vi "Test Filters.vi"() -> ()   [LabVIEW 2019]
uses:
  src/xy_utilities.lvlib
  src/subVIs/Zero Phase Lowpass Filter (multiple).vi
  src/subVIs/Savitsky Golay Weighted Filter (multiple).vi
  src/subVIs/Savitsky Golay Filter (multiple).vi
  src/subVIs/Moving Average (multiple).vi
panel:
  in  "cutoff period (data)":dbl
  in  "Window":dbl
  in  "Window Order":i32
  in  "polynomial order (3)":i32=3
  out "Intensity Graph 2":dbl[][](graph)
  out "Intensity Graph":dbl[][](graph)
  in  "side points":dbl
  in  "Dataset":T1(ring)=enum."superlattice waveguide"
  in  "index":i32
  out "XY Data Filtered 2":cluster{"X-array":dbl[], "Y-array":dbl[]}[](graph)
  in  "Filter":enum16{"Lowpass", "SG", "SGW", "Moving"}(ring)
  out "execution time (s)":dbl
  out "XY Data Filtered":cluster{"X-array":dbl[], "Y-array":dbl[]}[](graph)
  out "XY Data":cluster{"X-array":dbl[], "Y-array":dbl[]}[](graph)
  # "0: 21\"\n5: 0.09\""
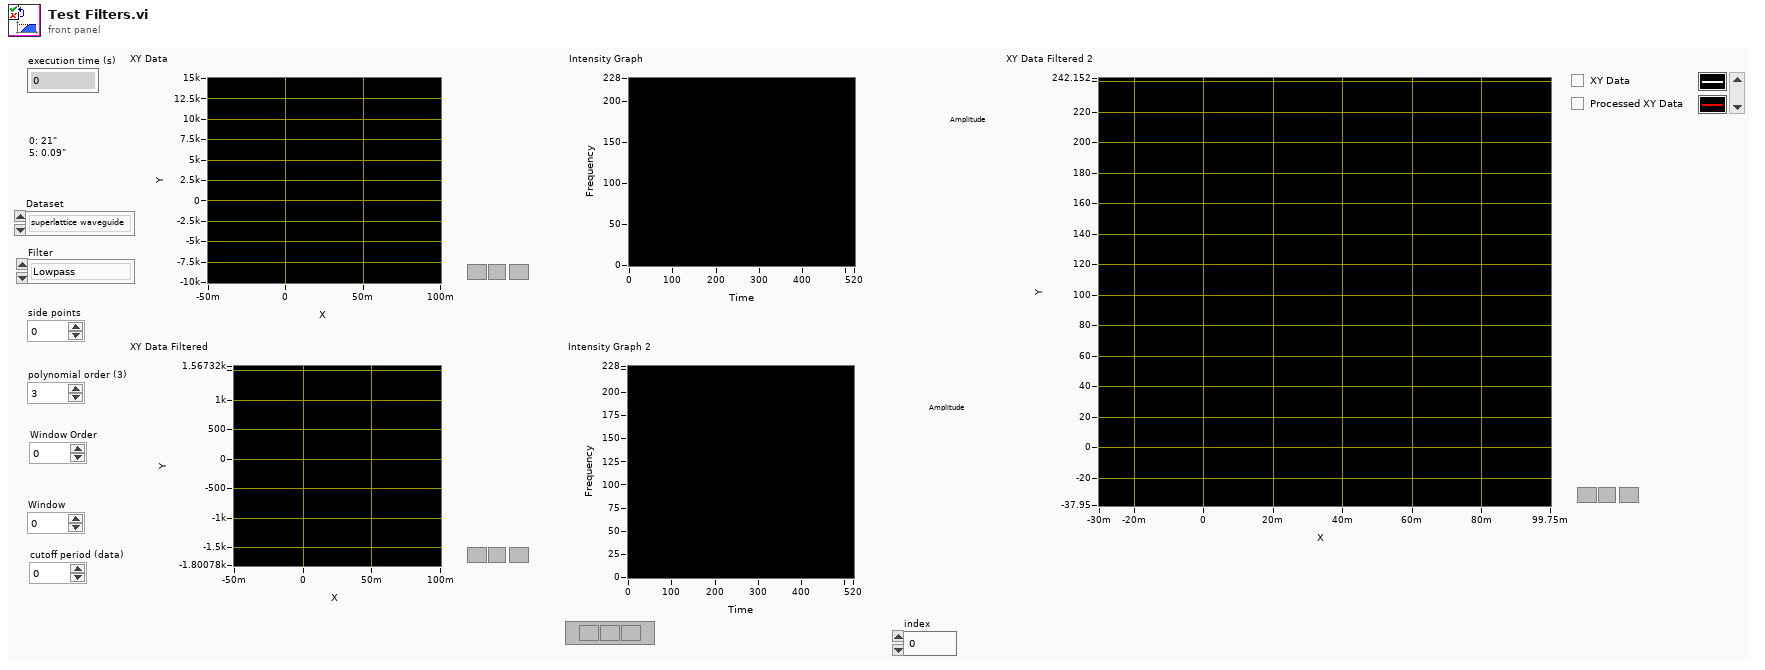
[diagram p1: front panel]
types:
  T1 = enum16{"thermal waveguide", "superlattice waveguide", "decay in atmosphere"}
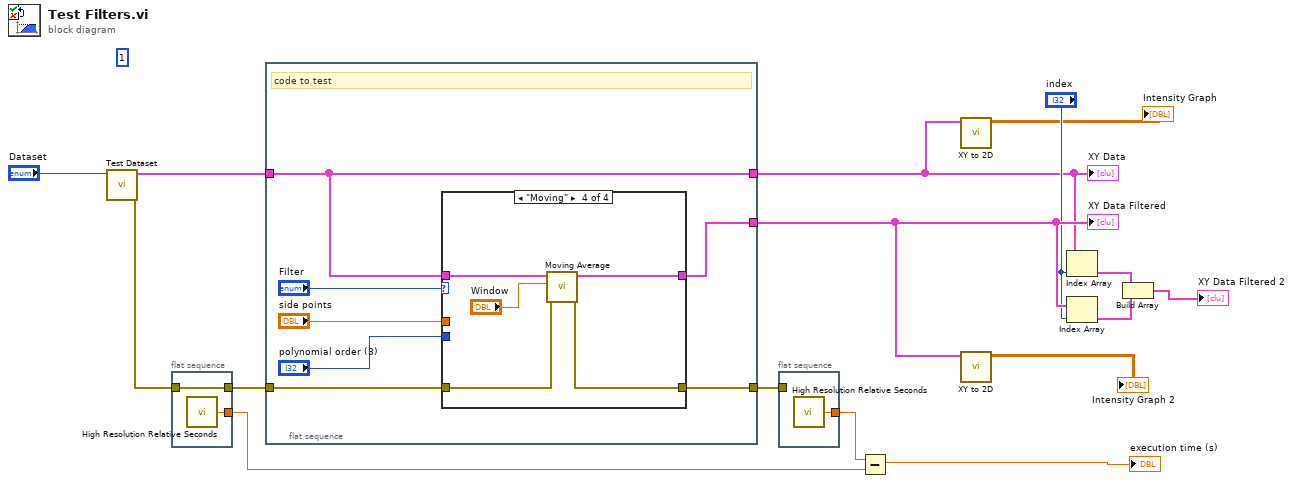
[diagram p0: block diagram]
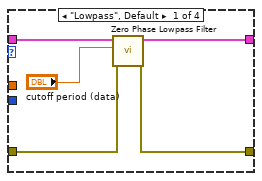
[diagram p2: hidden frame]
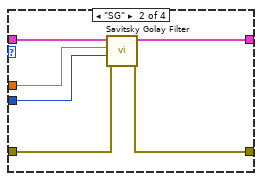
[diagram p3: hidden frame]
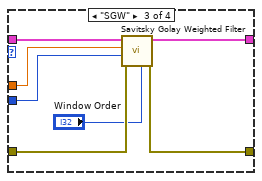
[diagram p4: hidden frame]
diagram:
  (unwired) 1
  n1 = call "Test Dataset.vi"("Enum"="Dataset") -> ("error out"=w16:errorcluster, "XY-data out"=w15:cluster{"X-array":dbl[], "Y-array":dbl[]}[])  [unwired: 8 in, 1 out]
  n2 = flat-sequence {
    tunnel: [w18] -> w5
    tunnel: w16 -> [w18]
    tunnel: [w17] -> w6
    frame #0 {
      n3 = call <vilib>:"High Resolution Relative Seconds.vi"() -> ("relative seconds"=w17:dbl)
    }
  }
  n4 = flat-sequence {
    tunnel: w15 -> [w25]
    tunnel: [w24] -> w13
    tunnel: w5 -> [w23]
    tunnel: [w22] -> w4
    tunnel: [w25] -> w3
    frame #0 {
      # "code to test"
      n5 = case shown="\"Moving\"" "Filter" {
        tunnel: w25 -> [w30 w36 w43 w48]
        tunnel: [w29 w35 w42 w47] -> w24
        tunnel: w23 -> [w28 w34 w41 w46]
        tunnel: [w27 w33 w40 w45] -> w22
        tunnel: "side points" -> [_ w32 w39 _]
        tunnel: "polynomial order (3)" -> [_ w31 w38 _]
        frame "Lowpass", Default {
          n6 = call-poly "Zero Phase Lowpass Filter.vi"("error in (no error)"=w28, "cutoff period (data)"="cutoff period (data)", "XY-data"=w30) -> ("error out"=w27:errorcluster, "XY-data out"=w29:cluster{"X-array":dbl[], "Y-array":dbl[]}[])  [unwired: 7 in]
        }
        frame "SG" {
          n7 = call-poly "Savitsky Golay Filter.vi"("error in (no error)"=w34, "polynomial order (3)"=w31, "side points (6)"=w32, "XY-data"=w36) -> ("error out"=w33:errorcluster, "XY-data out"=w35:cluster{"X-array":dbl[], "Y-array":dbl[]}[])  [unwired: 6 in]
        }
        frame "SGW" {
          n8 = call-poly "Savitsky Golay Weighted Filter.vi"("Window Order"="Window Order", "error in (no error)"=w41, "polynomial order (3)"=w38, "side points (6)"=w39, "XY-data"=w43) -> ("error out"=w40:errorcluster, "XY-data out"=w42:cluster{"X-array":dbl[], "Y-array":dbl[]}[])  [unwired: 5 in]
        }
        frame "Moving" {
          n9 = call-poly "Moving Average.vi"("error in (no error)"=w46, "Window"="Window", "XY-data"=w48) -> ("error out"=w45:errorcluster, "XY-data out"=w47:cluster{"X-array":dbl[], "Y-array":dbl[]}[])  [unwired: 7 in]
        }
      }
    }
  }
  n10 = flat-sequence {
    tunnel: [w49] -> w7
    tunnel: w4 -> [_]
    frame #0 {
      n11 = call <vilib>:"High Resolution Relative Seconds.vi"() -> ("relative seconds"=w49:dbl)
    }
  }
  n12 = Subtract(x=w7, y=w6) -> (x-y=→"execution time (s)":dbl)
  n13 = call "XY to 2D.vi"("XY-data"=w3) -> ("2D Z Array"=→"Intensity Graph":dbl[][])  [unwired: 7 in, 3 out]
  n14 = call "XY to 2D.vi"("XY-data"=w13) -> ("2D Z Array"=→"Intensity Graph 2":dbl[][])  [unwired: 7 in, 3 out]
  n15 = Index Array(array=w3, index="index") -> (element=w11:cluster{"X-array":dbl[], "Y-array":dbl[]})
  n16 = Index Array(array=w13, index="index") -> (element=w12:cluster{"X-array":dbl[], "Y-array":dbl[]})
  n17 = Build Array(w11, w12) -> (→"XY Data Filtered 2":cluster{"X-array":dbl[], "Y-array":dbl[]}[])
  "XY Data" <- w3
  "XY Data Filtered" <- w13
